vi "waitForClient.vi"(8 "error in (no error)":errorcluster, 11 "TCPServer in":refnum<class "TCPServer.lvclass">) -> (0 "error out":errorcluster, 1 "timeout":bool, 2 "remote address":string, 3 "TCPServer out":refnum<class "TCPServer.lvclass">)   [LabVIEW 2016, in "TCPServer.lvclass"]
uses:
  TCPServer.lvclass
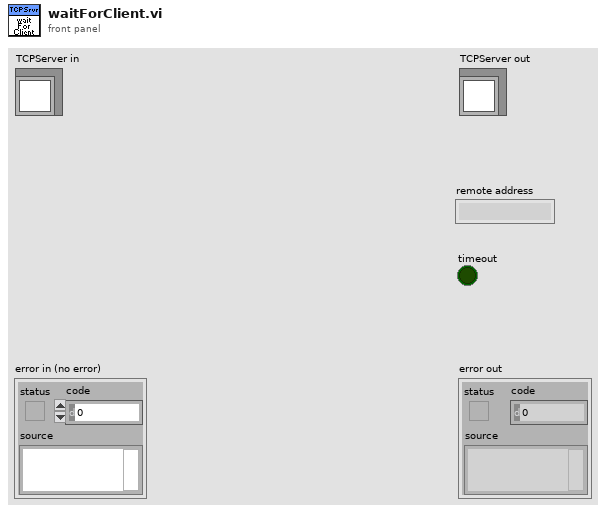
[diagram p1: front panel]
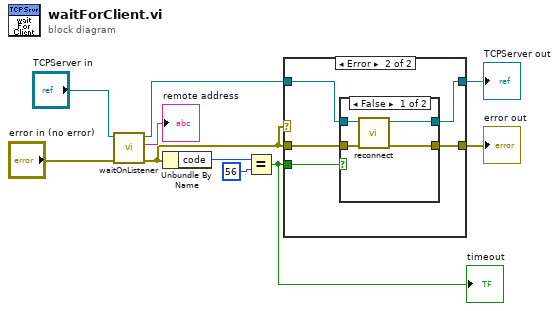
[diagram p0: block diagram]
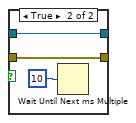
[diagram p3: hidden frame]
diagram:
  n1 = call "waitOnListener.vi"("error in (no error)"="error in (no error)", "TCPServer in"="TCPServer in") -> ("error out"=w2:errorcluster, "remote address"=→"remote address":string, "TCPServer out"=w5:refnum<class "TCPServer.lvclass">)  [unwired: 7 in]
  n2 = Unbundle By Name(w2) -> ("code"=w3:i32)
  n3 = Equal?(x=w3, y=56) -> (x = y?=w1:bool)
  "timeout" <- w1
  n4 = case shown="Error" w2 {
    tunnel: w5 -> [w12 w17]
    tunnel: [w12 w16] -> w10
    tunnel: w2 -> [w11 w15]
    tunnel: [w11 w14] -> w9
    tunnel: w1 -> [_ w13]
    frame No Error {
    }
    frame Error {
      n5 = case shown="False" w13 {
        tunnel: w17 -> [w21 w23]
        tunnel: [w20 w23] -> w16
        tunnel: w15 -> [w19 w22]
        tunnel: [w18 w22] -> w14
        frame False {
          n6 = call "reconnect.vi"("error in (no error)"=w19, "TCPServer in"=w21) -> ("error out"=w18:errorcluster, "TCPServer out"=w20:refnum<class "TCPServer.lvclass">)  [unwired: 8 in]
        }
        frame True {
          n7 = Wait Until Next ms Multiple(millisecond multiple=u32 10) -> ()  [unwired: 1 out]
        }
      }
    }
  }
  "error out" <- w9
  "TCPServer out" <- w10
